vi "run.vi"() -> ()   [LabVIEW 2016]
uses:
  <vilib>/addons/_JKI Toolkits/Caraya/classes/Test Result/Node Results.ctl
  <vilib>/addons/_JKI Toolkits/Caraya/classes/Test Result/Test Node.ctl
  <vilib>/addons/_JKI Toolkits/Caraya/classes/Test Result/Test Registration Data.ctl
  <vilib>/addons/_JKI Toolkits/Caraya/classes/Test Result/Assert Event Data.ctl
  <vilib>/addons/_JKI Toolkits/Caraya/classes/Test Runner.Folder/Test Runner.Folder.lvclass
  C:/Program Files/National Instruments/LabVIEW 2016/vi.lib/addons/_JKI Toolkits/Caraya/classes/Test Runner/Test Runner.lvclass
  <vilib>/addons/_JKI Toolkits/Caraya/classes/Test Result/Test Result.lvclass
  <vilib>/addons/_JKI Toolkits/Caraya/classes/Test Runner/Test Runner.lvclass
panel:
  out "Test Results":T1[](array[typedef])
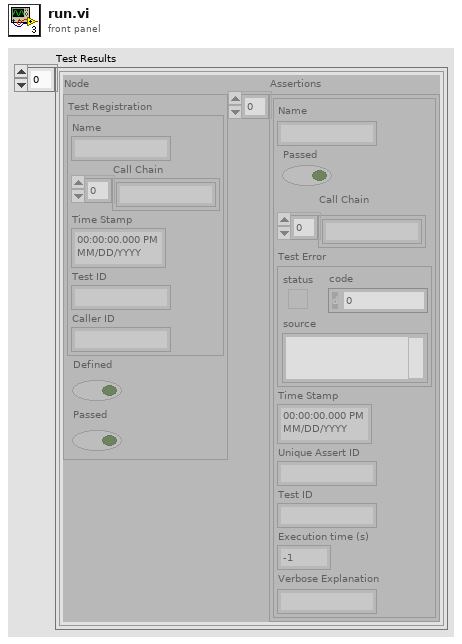
[diagram p1: front panel]
types:
  T1 = typedef "Caraya.lvlib/Test Result.lvclass/Node Results.ctl" = cluster{"Node":T2, "Assertions":T4[]}
  T2 = typedef "Caraya.lvlib/Test Result.lvclass/Test Node.ctl" = cluster{"Test Registration":T3, "Defined":bool, "Passed":bool}
  T3 = typedef "Caraya.lvlib/Test Result.lvclass/Test Registration Data.ctl" = cluster{"Name":string, "Call Chain":string[], "Time Stamp":timestamp, "Test ID":string, "Caller ID":string}
  T4 = typedef "Caraya.lvlib/Test Result.lvclass/Assert Event Data.ctl" = cluster{"Name":string, "Passed":bool, "Call Chain":string[], "Test Error":errorcluster, "Time Stamp":timestamp, "Unique Assert ID":string, "Test ID":string, "Execution time (s)":dbl, "Verbose Explanation":string}
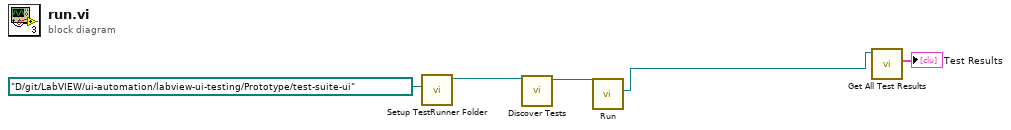
[diagram p0: block diagram]
diagram:
  n1 = call <vilib>:"Setup TestRunner Folder.vi"("Directory to search"=path "D:/git/LabVIEW/ui-automation/labview-ui-testing/Prototype/test-suite-ui") -> ("Test Runner.Folder out"=w2:refnum<class "Test Runner.Folder.lvclass">)  [unwired: 9 in, 1 out]
  n2 = call <vilib>:"Discover Tests.vi"("Test Runner in"=w2) -> ("Test Runner out"=w4:refnum<class "Test Runner.Folder.lvclass">)  [unwired: 9 in, 1 out]
  n3 = call <vilib>:"Run.vi"("Test Runner in"=w4) -> ("Test Suite Results"=w3:refnum<class "Test Result.lvclass">)  [unwired: 8 in, 2 out]
  n4 = call <vilib>:"Get All Test Results.vi"("Test Result in"=w3) -> ("Test Results"=→"Test Results":T1[])  [unwired: 8 in, 2 out]
